vi "ImagesCleanUp.vi"(9 "Pictures in":string[](array[string]), 10 "Team":string) -> (1 "Pictures out":string[](array[string]))   [LabVIEW 2017]
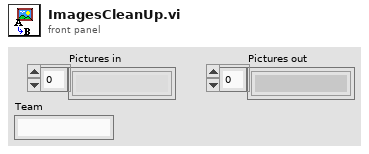
[diagram p1: front panel]
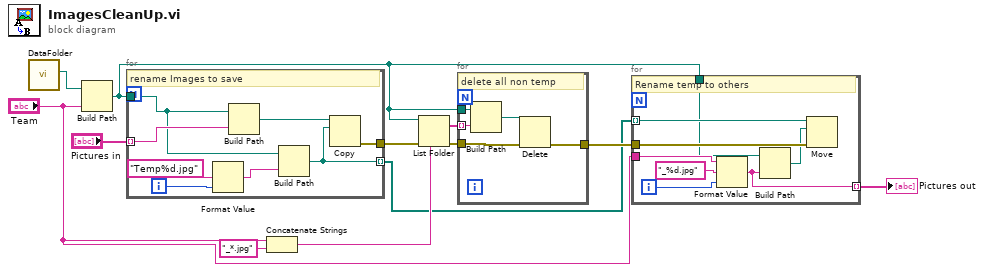
[diagram p0: block diagram]
diagram:
  n1 = call "DataFolder.vi"() -> ("appended path"=w11:path)  [unwired: 11 in]
  n2 = Build Path(base path=w11, name or relative path="Team") -> (appended path=w1:path)
  n3 = for {
    tunnel: "Pictures in" -> [w20] mode=indexing
    tunnel: w1 -> [w18]
    tunnel: [w14] -> w8
    tunnel: [w13] -> w4 mode=indexing
    i -> [w17]
    # "rename Images to save"
    n4 = Format Value(format string="Temp%d.jpg", value (0)=w17) -> (output string=w15:string)  [unwired: 1 in]
    n5 = Build Path(base path=w18, name or relative path=w20) -> (appended path=w19:path)
    n6 = Build Path(base path=w18, name or relative path=w15) -> (appended path=w13:path)
    n7 = Copy(10:w13, 11:w19) -> (0:w14:errorcluster)  [unwired: 3 in, 2 out]
  }
  n8 = Concatenate Strings("Team", "_*.jpg" ("string")) -> (w9:string)
  n9 = List Folder(path=w1, pattern=w9, error in=w8) -> (filenames=w6:string[], error out=w7:errorcluster)  [unwired: 1 in, 2 out]
  n10 = for {
    tunnel: w7 -> [w25]
    tunnel: w1 -> [w23]
    tunnel: w6 -> [w22] mode=indexing
    tunnel: [w21] -> w5
    # "delete all non temp"
    n11 = Build Path(base path=w23, name or relative path=w22) -> (appended path=w24:path)
    n12 = Delete(path (use dialog)=w24, error in=w25) -> (error out=w21:errorcluster)  [unwired: 3 in, 2 out]
  }
  n13 = for {
    tunnel: w5 -> [w33]
    tunnel: w4 -> [w32] mode=indexing
    tunnel: w1 -> [w27]
    tunnel: "Team" -> [w30]
    tunnel: [w26] -> w2 mode=indexing
    i -> [w29]
    # "Rename temp to others"
    n14 = Format Value(string ("")=w30, format string="_%d.jpg", value (0)=w29) -> (output string=w26:string)
    n15 = Build Path(base path=w27, name or relative path=w26) -> (appended path=w28:path)
    n16 = Move(source path=w32, error in=w33, 10:w28) -> ()  [unwired: 2 in, 3 out]
  }
  "Pictures out" <- w2
